vi "Set_Rain_CupSize.vi"(1 "Rain cup size":i16) -> (0 "Succes?":bool)   [LabVIEW 2013]
uses:
  VantagePro.dll
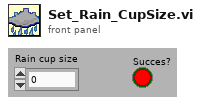
[diagram p1: front panel]
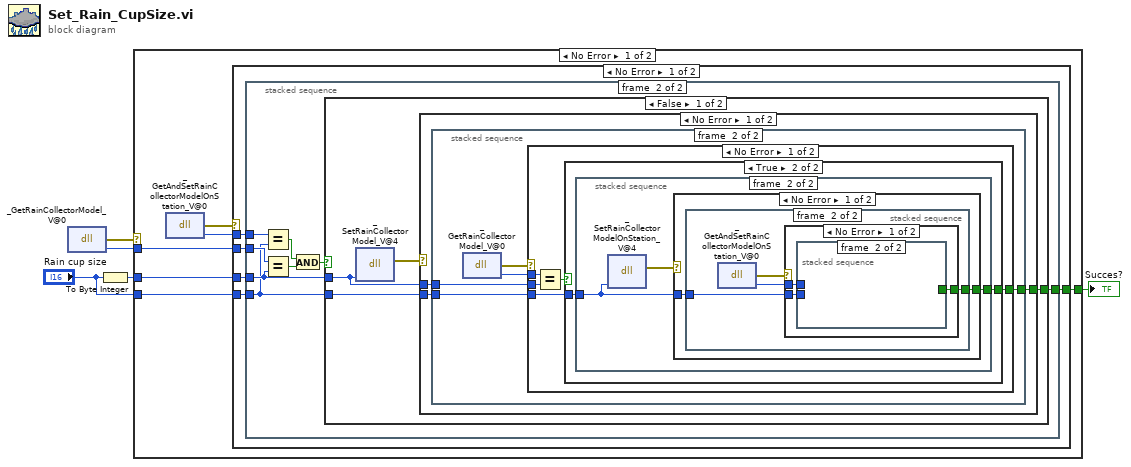
[diagram p0: block diagram]
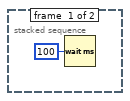
[diagram p2: hidden frame]
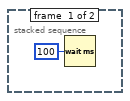
[diagram p3: hidden frame]
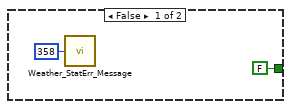
[diagram p4: hidden frame]
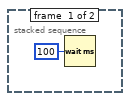
[diagram p5: hidden frame]
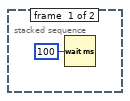
[diagram p6: hidden frame]
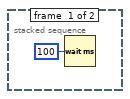
[diagram p7: hidden frame]
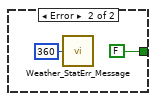
[diagram p8: hidden frame]
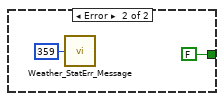
[diagram p9: hidden frame]
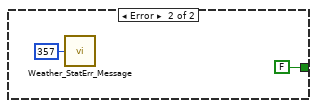
[diagram p10: hidden frame]
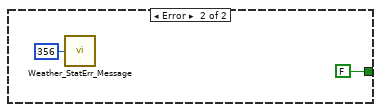
[diagram p11: hidden frame]
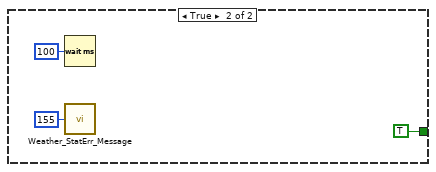
[diagram p12: hidden frame]
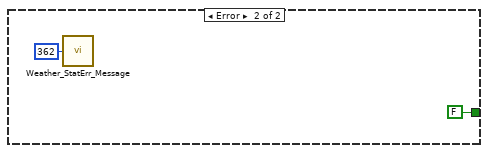
[diagram p13: hidden frame]
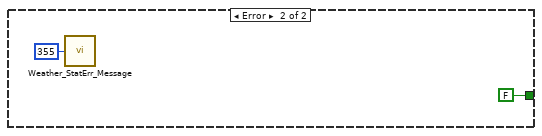
[diagram p14: hidden frame]
diagram:
  n1 = dll-call lib="C:/Users/Bob van Eijk/Desktop/LabView Projects 13/HiSPARC Weather Station/Develop/VantagePro.dll" fn="_GetRainCollectorModel_V@0" label="Get Rain Collector"() -> (error out=w2:errorcluster, "return type"=w1:i8)  [unwired: 3 in, 1 out]
  n2 = To Byte Integer(number="Rain cup size") -> (8bit integer=w5:i8)
  n3 = case shown="No Error" w2 {
    tunnel: w5 -> [w11 _]
    tunnel: "Rain cup size" -> [w10 _]
    tunnel: [w9 FALSE] -> w3
    tunnel: w1 -> [w8 _]
    frame No Error {
      n4 = dll-call lib="C:/Users/Bob van Eijk/Desktop/LabView Projects 13/HiSPARC Weather Station/Develop/VantagePro.dll" fn="_GetAndSetRainCollectorModelOnStation_V@0" label="Get Rain Collector\nfrom Station"() -> (error out=w7:errorcluster, "return type"=w6:i16)  [unwired: 3 in, 1 out]
      n5 = case shown="No Error" w7 {
        tunnel: w11 -> [w16 _]
        tunnel: w10 -> [w15 _]
        tunnel: [w14 FALSE] -> w9
        tunnel: w8 -> [w13 _]
        tunnel: w6 -> [w12 _]
        frame No Error {
          n6 = stacked-sequence {
            tunnel: w16 -> [_ w24]
            tunnel: w15 -> [_ w20]
            tunnel: [_ w25] -> w14
            tunnel: w13 -> [_ w23]
            tunnel: w12 -> [_ w19]
            frame #0 {
              n7 = Wait (ms)(milliseconds to wait=u32 100) -> ()  [unwired: 1 out]
            }
            frame #1 {
              n8 = Equal?(x=w19, y=w20) -> (x = y?=w18:bool)
              n9 = Equal?(x=w23, y=w24) -> (x = y?=w21:bool)
              n10 = And(x=w18, y=w21) -> (x .and. y?=w22:bool)
              n11 = case shown="False" w22 {
                tunnel: w20 -> [w29 _]
                tunnel: [w27 TRUE] -> w25
                tunnel: w24 -> [w26 _]
                frame False {
                  n12 = dll-call lib="C:/Users/Bob van Eijk/Desktop/LabView Projects 13/HiSPARC Weather Station/Develop/VantagePro.dll" fn="_SetRainCollectorModel_V@4" label="Set Rain Collector"("RainCollectorModel"=w26) -> (error out=w28:errorcluster)  [unwired: 5 in, 1 out]
                  n13 = case shown="No Error" w28 {
                    tunnel: [w30 FALSE] -> w27
                    tunnel: w26 -> [w32 _]
                    tunnel: w29 -> [w31 _]
                    frame No Error {
                      n14 = stacked-sequence {
                        tunnel: w32 -> [_ w37]
                        tunnel: w31 -> [_ w36]
                        tunnel: [_ w34] -> w30
                        frame #0 {
                          n15 = Wait (ms)(milliseconds to wait=u32 100) -> ()  [unwired: 1 out]
                        }
                        frame #1 {
                          n16 = dll-call lib="C:/Users/Bob van Eijk/Desktop/LabView Projects 13/HiSPARC Weather Station/Develop/VantagePro.dll" fn="_GetRainCollectorModel_V@0" label="Get Rain Collector"() -> (error out=w35:errorcluster, "return type"=w38:i8)  [unwired: 3 in, 1 out]
                          n17 = case shown="No Error" w35 {
                            tunnel: [w43 FALSE] -> w34
                            tunnel: w38 -> [w42 _]
                            tunnel: w37 -> [w41 _]
                            tunnel: w36 -> [w39 _]
                            frame No Error {
                              n18 = Equal?(x=w42, y=w41) -> (x = y?=w40:bool)
                              n19 = case shown="True" w40 {
                                tunnel: [FALSE w47] -> w43
                                tunnel: w39 -> [_ w46]
                                frame False {
                                n20 = call "Weather_StatErr_Message.vi"("Message number"=358) -> ()  [unwired: 1 out]
                                }
                                frame True {
                                n21 = stacked-sequence {
                                tunnel: [_ w51] -> w47
                                tunnel: w46 -> [_ w50]
                                frame #0 {
                                n22 = Wait (ms)(milliseconds to wait=u32 100) -> ()  [unwired: 1 out]
                                }
                                frame #1 {
                                n23 = dll-call lib="C:/Users/Bob van Eijk/Desktop/LabView Projects 13/HiSPARC Weather Station/Develop/VantagePro.dll" fn="_SetRainCollectorModelOnStation_V@4" label="Set Rain Collector\non Station"("rainCModel"=w50) -> (error out=w49:errorcluster)  [unwired: 4 in, 2 out]
                                n24 = case shown="No Error" w49 {
                                tunnel: w50 -> [w53 _]
                                tunnel: [w52 FALSE] -> w51
                                frame No Error {
                                n25 = stacked-sequence {
                                tunnel: w53 -> [_ w57]
                                tunnel: [_ w55] -> w52
                                frame #0 {
                                n26 = Wait (ms)(milliseconds to wait=u32 100) -> ()  [unwired: 1 out]
                                }
                                frame #1 {
                                n27 = dll-call lib="C:/Users/Bob van Eijk/Desktop/LabView Projects 13/HiSPARC Weather Station/Develop/VantagePro.dll" fn="_GetAndSetRainCollectorModelOnStation_V@0" label="Get Rain Collector\nfrom Station"() -> (error out=w58:errorcluster, "return type"=w56:i16)  [unwired: 3 in, 1 out]
                                n28 = case shown="No Error" w58 {
                                tunnel: w57 -> [w61 _]
                                tunnel: w56 -> [w60 _]
                                tunnel: [w59 FALSE] -> w55
                                frame No Error {
                                n29 = stacked-sequence {
                                tunnel: w61 -> [_ w66]
                                tunnel: w60 -> [_ w65]
                                tunnel: [_ w63] -> w59
                                frame #0 {
                                n30 = Wait (ms)(milliseconds to wait=u32 100) -> ()  [unwired: 1 out]
                                }
                                frame #1 {
                                n31 = Equal?(x=w65, y=w66) -> (x = y?=w64:bool)
                                n32 = case shown="True" w64 {
                                tunnel: [FALSE TRUE] -> w63
                                frame False {
                                n33 = call "Weather_StatErr_Message.vi"("Message number"=361) -> ()  [unwired: 1 out]
                                }
                                frame True {
                                n34 = call "Weather_StatErr_Message.vi"("Message number"=255) -> ()  [unwired: 1 out]
                                }
                                }
                                }
                                }
                                }
                                frame Error {
                                n35 = call "Weather_StatErr_Message.vi"("Message number"=360) -> ()  [unwired: 1 out]
                                }
                                }
                                }
                                }
                                }
                                frame Error {
                                n36 = call "Weather_StatErr_Message.vi"("Message number"=359) -> ()  [unwired: 1 out]
                                }
                                }
                                }
                                }
                                }
                              }
                            }
                            frame Error {
                              n37 = call "Weather_StatErr_Message.vi"("Message number"=357) -> ()  [unwired: 1 out]
                            }
                          }
                        }
                      }
                    }
                    frame Error {
                      n38 = call "Weather_StatErr_Message.vi"("Message number"=356) -> ()  [unwired: 1 out]
                    }
                  }
                }
                frame True {
                  n39 = Wait (ms)(milliseconds to wait=u32 100) -> ()  [unwired: 1 out]
                  n40 = call "Weather_StatErr_Message.vi"("Message number"=155) -> ()  [unwired: 1 out]
                }
              }
            }
          }
        }
        frame Error {
          n41 = call "Weather_StatErr_Message.vi"("Message number"=362) -> ()  [unwired: 1 out]
        }
      }
    }
    frame Error {
      n42 = call "Weather_StatErr_Message.vi"("Message number"=355) -> ()  [unwired: 1 out]
    }
  }
  "Succes?" <- w3
